vi "hpanel_set_xy_graph_properties.vi"(11 "hydraharp_panel in":refnum<class "hydraharp_panel.lvclass">) -> ()   [LabVIEW 2015, in "hydraharp_panel.lvclass"]
uses:
  hydraharp_panel.lvclass
  UI/panel_class/panel.lvclass/panel.ctl
  UI/panel_class/panel.lvclass
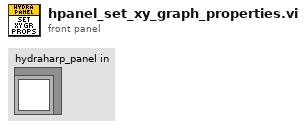
[diagram p1: front panel]
types:
  T1 = typedef "ui_plot_references.ctl" = cluster{"plots":refnum<vi>, "chart":refnum<vi>, "graph":refnum<vi>, "map":refnum<vi>, "XY Graph":refnum<vi>}
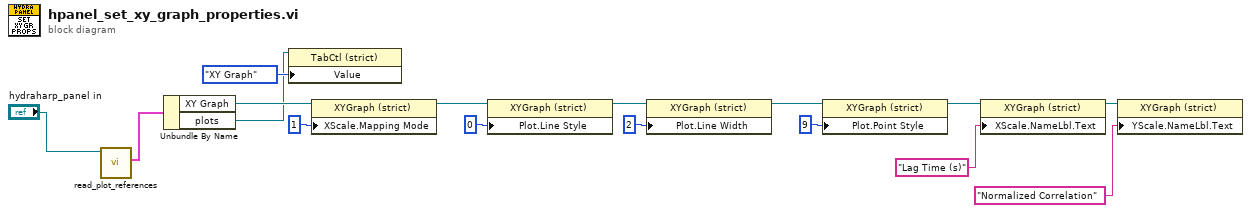
[diagram p0: block diagram]
diagram:
  n1 = call "read_plot_references.vi"("panel in"="hydraharp_panel in") -> ("plot_references"=w1:T1)  [unwired: 8 in, 2 out]
  n2 = Unbundle By Name(w1) -> ("XY Graph"=w13:refnum<vi>, "plots"=w11:refnum<vi>)
  n3 = property class="TabCtl (strict)"(reference=w11, "Value"=enum32{"Chart", "Graph", "Map", "XY Graph"}."XY Graph") -> ()  [unwired: 1 in, 2 out]
  n4 = property class="XYGraph (strict)"(reference=w13, "XScale.Mapping Mode"=u8 1 ("X Scale.Mapping Mode")) -> (reference out=w15:refnum<vi>)  [unwired: 1 in, 1 out]
  n5 = property class="XYGraph (strict)"(reference=w15, "Plot.Line Style"=u8 0) -> (reference out=w6:refnum<vi>)  [unwired: 1 in, 1 out]
  n6 = property class="XYGraph (strict)"(reference=w6, "Plot.Line Width"=u8 2) -> (reference out=w5:refnum<vi>)  [unwired: 1 in, 1 out]
  n7 = property class="XYGraph (strict)"(reference=w5, "Plot.Point Style"=u8 9) -> (reference out=w4:refnum<vi>)  [unwired: 1 in, 1 out]
  n8 = property class="XYGraph (strict)"(reference=w4, "XScale.NameLbl.Text"="Lag Time (s)" ("X Scale.Name Label.Text")) -> (reference out=w9:refnum<vi>)  [unwired: 1 in, 1 out]
  n9 = property class="XYGraph (strict)"(reference=w9, "YScale.NameLbl.Text"="Normalized Correlation" ("Y Scale.Name Label.Text")) -> ()  [unwired: 1 in, 2 out]
